vi "PreUninstall.vi"(10 "Variant":variant) -> (0 "error out":errorcluster)   [LabVIEW 2012]
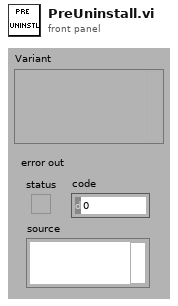
[diagram p1: front panel]
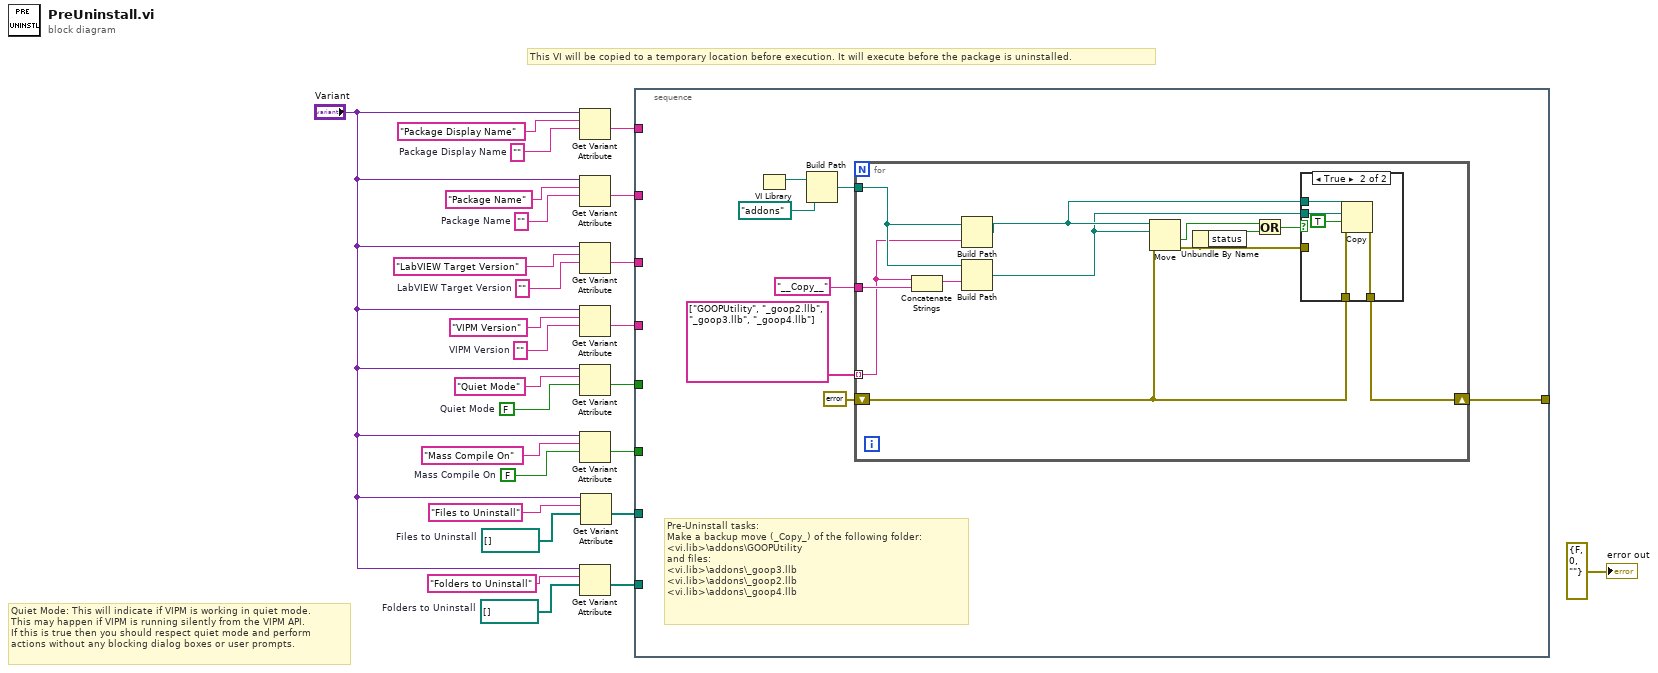
[diagram p0: block diagram]
diagram:
  w3 = path[] []  # Folders to Uninstall
  w7 = path[] []  # Files to Uninstall
  w8 = FALSE  # Mass Compile On
  w9 = ""  # Package Display Name
  w16 = FALSE  # Quiet Mode
  w19 = ""  # VIPM Version
  w21 = ""  # LabVIEW Target Version
  w23 = ""  # Package Name
  # "Quiet Mode: This will indicate if VIPM is working in quiet mode.\nThis may happen if VIPM is running silently from the VIPM API.\nIf this is true then you should respect quiet mode and perform\nactions without any blocking dialog boxes or user prompts."
  # "This VI will be copied to a temporary location before execution. It will execute before the package is uninstalled."
  n1 = Get Variant Attribute(Variant="Variant", name="Package Display Name", default value (empty Variant)=w9) -> (value=w15:string)  [unwired: 1 in, 3 out]
  n2 = Get Variant Attribute(Variant="Variant", name="Package Name", default value (empty Variant)=w23) -> (value=w14:string)  [unwired: 1 in, 3 out]
  n3 = Get Variant Attribute(Variant="Variant", name="LabVIEW Target Version", default value (empty Variant)=w21) -> (value=w13:string)  [unwired: 1 in, 3 out]
  n4 = Get Variant Attribute(Variant="Variant", name="VIPM Version", default value (empty Variant)=w19) -> (value=w12:string)  [unwired: 1 in, 3 out]
  n5 = Get Variant Attribute(Variant="Variant", name="Quiet Mode", default value (empty Variant)=w16) -> (value=w11:bool)  [unwired: 1 in, 3 out]
  n6 = Get Variant Attribute(Variant="Variant", name="Mass Compile On", default value (empty Variant)=w8) -> (value=w10:bool)  [unwired: 1 in, 3 out]
  n7 = Get Variant Attribute(Variant="Variant", name="Folders to Uninstall", default value (empty Variant)=w3) -> (value=w2:path[])  [unwired: 1 in, 3 out]
  n8 = Get Variant Attribute(Variant="Variant", name="Files to Uninstall", default value (empty Variant)=w7) -> (value=w5:path[])  [unwired: 1 in, 3 out]
  n9 = stacked-sequence {
    tunnel: w15 -> [_]
    tunnel: w14 -> [_]
    tunnel: w13 -> [_]
    tunnel: w12 -> [_]
    tunnel: w11 -> [_]
    tunnel: w10 -> [_]
    tunnel: w5 -> [_]
    tunnel: w2 -> [_]
    tunnel: [w27] -> _
    frame #0 {
      # "Pre-Uninstall tasks:\nMake a backup move (_Copy_) of the following folder:\n<vi.lib>\\addons\\GOOPUtility\nand files:\n<vi.lib>\\addons\\_goop3.llb\n<vi.lib>\\addons\\_goop2.llb\n<vi.lib>\\addons\\_goop4.llb"
      n10 = VI Library() -> (path=w30:path)
      n11 = Build Path(base path=w30, name or relative path=path "addons" ("path")) -> (appended path=w32:path)
      n12 = for {
        tunnel: "__Copy__" ("name or relative path") -> [w40]
        tunnel: w32 -> [w38]
        tunnel: string[] ["GOOPUtility", "_goop2.llb", "_goop3.llb", "_goop4.llb"] -> [w37] mode=indexing
        shift-right: [w35] -> w27
        shift-left: errorcluster {"status"=FALSE, "code"=0, "source"=""} ("error out") -> [w36]
        n13 = Concatenate Strings(w37, w40) -> (w39:string)
        n14 = Build Path(base path=w38, name or relative path=w37) -> (appended path=w42:path)
        n15 = Build Path(base path=w38, name or relative path=w39) -> (appended path=w34:path)
        n16 = Move(source path=w42, error in=w36, 10:w34) -> (error out=w41:errorcluster, 1:w44:bool)  [unwired: 2 in, 1 out]
        n17 = Unbundle By Name(w41) -> ("status"=w45:bool)
        n18 = Or(x=w44, y=w45) -> (x .or. y?=w43:bool)
        n19 = case shown="True" w43 {
          tunnel: w42 -> [_ w51]
          tunnel: w34 -> [_ w50]
          tunnel: w41 -> [w46 _]
          tunnel: [w46 w48] -> w35
          tunnel: w36 -> [_ w47]
          frame False {
          }
          frame True {
            n20 = Copy(8:w47, 9:TRUE ("overwrite (F)"), 10:w50, 11:w51) -> (0:w48:errorcluster)  [unwired: 1 in, 2 out]
          }
        }
      }
    }
  }
  "error out" <- errorcluster {"status"=FALSE, "code"=0, "source"=""} ("error out")
